vi "add delta range(SubVI).vi"(10 "字符串":string) -> (1 "ok or cancel":bool, 2 "连接的字符串":string)   [LabVIEW 2019, in "Add Seq.lvlib"]
uses:
  Add Seq.lvlib
  lib/Keithley 622x/Configure/2182 -A/Low Level/Typedefs/KE2182 -- Voltage Ranges.ctl
  lib/Keithley 622x/Keithley 622x.lvlib
panel:
  in  "Man / Selected\nRange":T1
  in  "cancel":bool
  in  "ok":bool
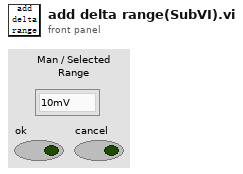
[diagram p1: front panel]
types:
  T1 = typedef "Keithley 622x.lvlib/KE2182 -- Voltage Ranges.ctl" = enum16{"10mV", "100mV", "1V", "10V", "100V"}
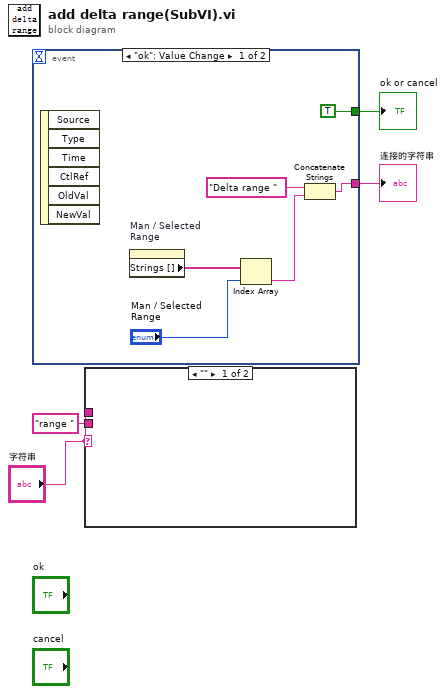
[diagram p0: block diagram]
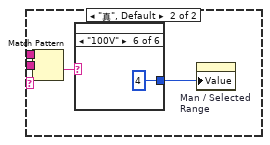
[diagram p2: hidden frame]
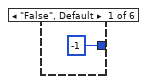
[diagram p3: hidden frame]
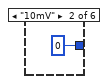
[diagram p4: hidden frame]
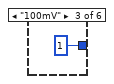
[diagram p5: hidden frame]
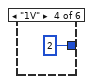
[diagram p6: hidden frame]
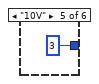
[diagram p7: hidden frame]
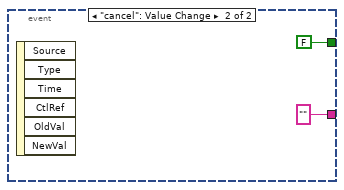
[diagram p8: hidden frame]
diagram:
  n1 = event shown="[0] \"ok\": Value Change" {
    selector: _ -> [_ _]
    dyn-events: _ -> [_ _]
    timeout: _ -> [_ _]
    tunnel: [TRUE FALSE] -> w4
    tunnel: [w8 "" ("分隔符")] -> w3
    event "ok": Value Change {
      n2 = event-data() -> ()  [unwired: 1 in, 6 out]
      n3 = property on="Man / Selected\nRange" class="Enum (strict)"() -> ("Strings []"=w7:string[])  [unwired: 2 in, 2 out]
      n4 = Index Array(array=w7, index="Man / Selected\nRange") -> (element=w5:string)
      n5 = Concatenate Strings("Delta range " ("字符串"), w5) -> (w8:string)
    }
    event "cancel": Value Change {
      n6 = event-data() -> ()  [unwired: 1 in, 6 out]
    }
  }
  "ok or cancel" <- w4
  "连接的字符串" <- w3
  n7 = case shown="\"\"" "字符串" {
    tunnel: "字符串" -> [_ w16]
    tunnel: "range " ("regular expression") -> [_ w15]
    frame "" {
    }
    frame "真", Default {
      n8 = Match Pattern(string=w16, regular expression=w15) -> (after substring=w14:string)  [unwired: 1 in, 3 out]
      n9 = case shown="\"100V\"" w14 {
        tunnel: [-1 0 1 2 3 4] -> w13
        frame "False", Default {
        }
        frame "10mV" {
        }
        frame "100mV" {
        }
        frame "1V" {
        }
        frame "10V" {
        }
        frame "100V" {
        }
      }
      n10 = property on="Man / Selected\nRange" class="Enum (strict)"("Value"=w13) -> ()  [unwired: 2 in, 2 out]
    }
  }
